vi "DataCapNew.vi"() -> ()   [LabVIEW 2022 SP3]
uses:
  b4946857-5c5e-463d-9afd-b13ad1e40e0e.vi
  37c4a671-fe09-4c27-8638-ee31c478114f.vi
  <vilib>/Analysis/baseanly.llb/Mean (DBL).vi
  <vilib>/ULx/Create Channel.llb/ULx Create Channel (AI-Voltage-Basic).vi
  <vilib>/ULx/Timing.llb/ULx Timing (Sample Clock).vi
  <vilib>/ULx/Read.llb/ULx Read (Analog 1D Wfm NChan NSamp).vi
  <vilib>/Waveform/WDTOps.llb/WDT Number of Waveform Samples DBL.vi
  <vilib>/Waveform/WDTFileIO.llb/Export Waveforms To Spreadsheet File (1D).vi
  <vilib>/Instr/_visa.llb/VISA Configure Serial Port (Instr).vi
  <vilib>/ptbypt/NI_PtbyPt.lvlib
  <vilib>/Analysis/NI_AALBase.lvlib
panel:
  out "Drag Chart":dbl(graph)
  out "Moving Average Size":dbl
  in  "sample length":i32=100
  out "Lift Chart":dbl(graph)
  out "DAQ Samples":i32
  out "DAQ Voltage Data":waveform(dbl)[](graph)
  in  "Samples":i32=-1
  in  "Sample Rate":dbl=1000.0
  in  "Manual Size":dbl
  out "Serial Samples":dbl
  in  "GoTo Angle":dbl
  out "read buffer":string
  in  "Send":bool
  in  "Period":dbl
  in  "Max Angle":dbl min=-359.9999 max=359.9999
  in  "Command":u16(ring) items=["Send Max Angle", "Send Period", "Stop Movement", "Start Movement", "Sinusoidal Motion", "Go forward", "Go backwards", "Linear Ramp", "GoTo Angle", "Set Manual Movement Size"]
  out "Angle":dbl
  in  "Port":refnum<visa-resource-name>
  out "Angle Meter":dbl(knob) scale=-100.0..100.0 scale format="%#_2f"
  out "Angle Chart":dbl(graph)
  in  "Set zero":bool
  in  "Port 2":refnum<visa-resource-name>
  out "ENC Chart 2":dbl(graph)
  out "ENC 2":dbl
  out "ENC Meter 2":dbl(knob) scale=-100.0..100.0 scale format="%#_2f"
  in  "Serial CSV Path":path
  out "Data written Serial":dbl
  out "Data written ENC":dbl
  out "Boolean 3":bool
  in  "DAQ":bool
  out "Boolean 2":bool
  in  "ENC":bool
  out "Boolean":bool
  in  "Serial":bool
  in  "STOP":bool
  # "Serial Motor Control"
  # "Serial Encoder Readout"
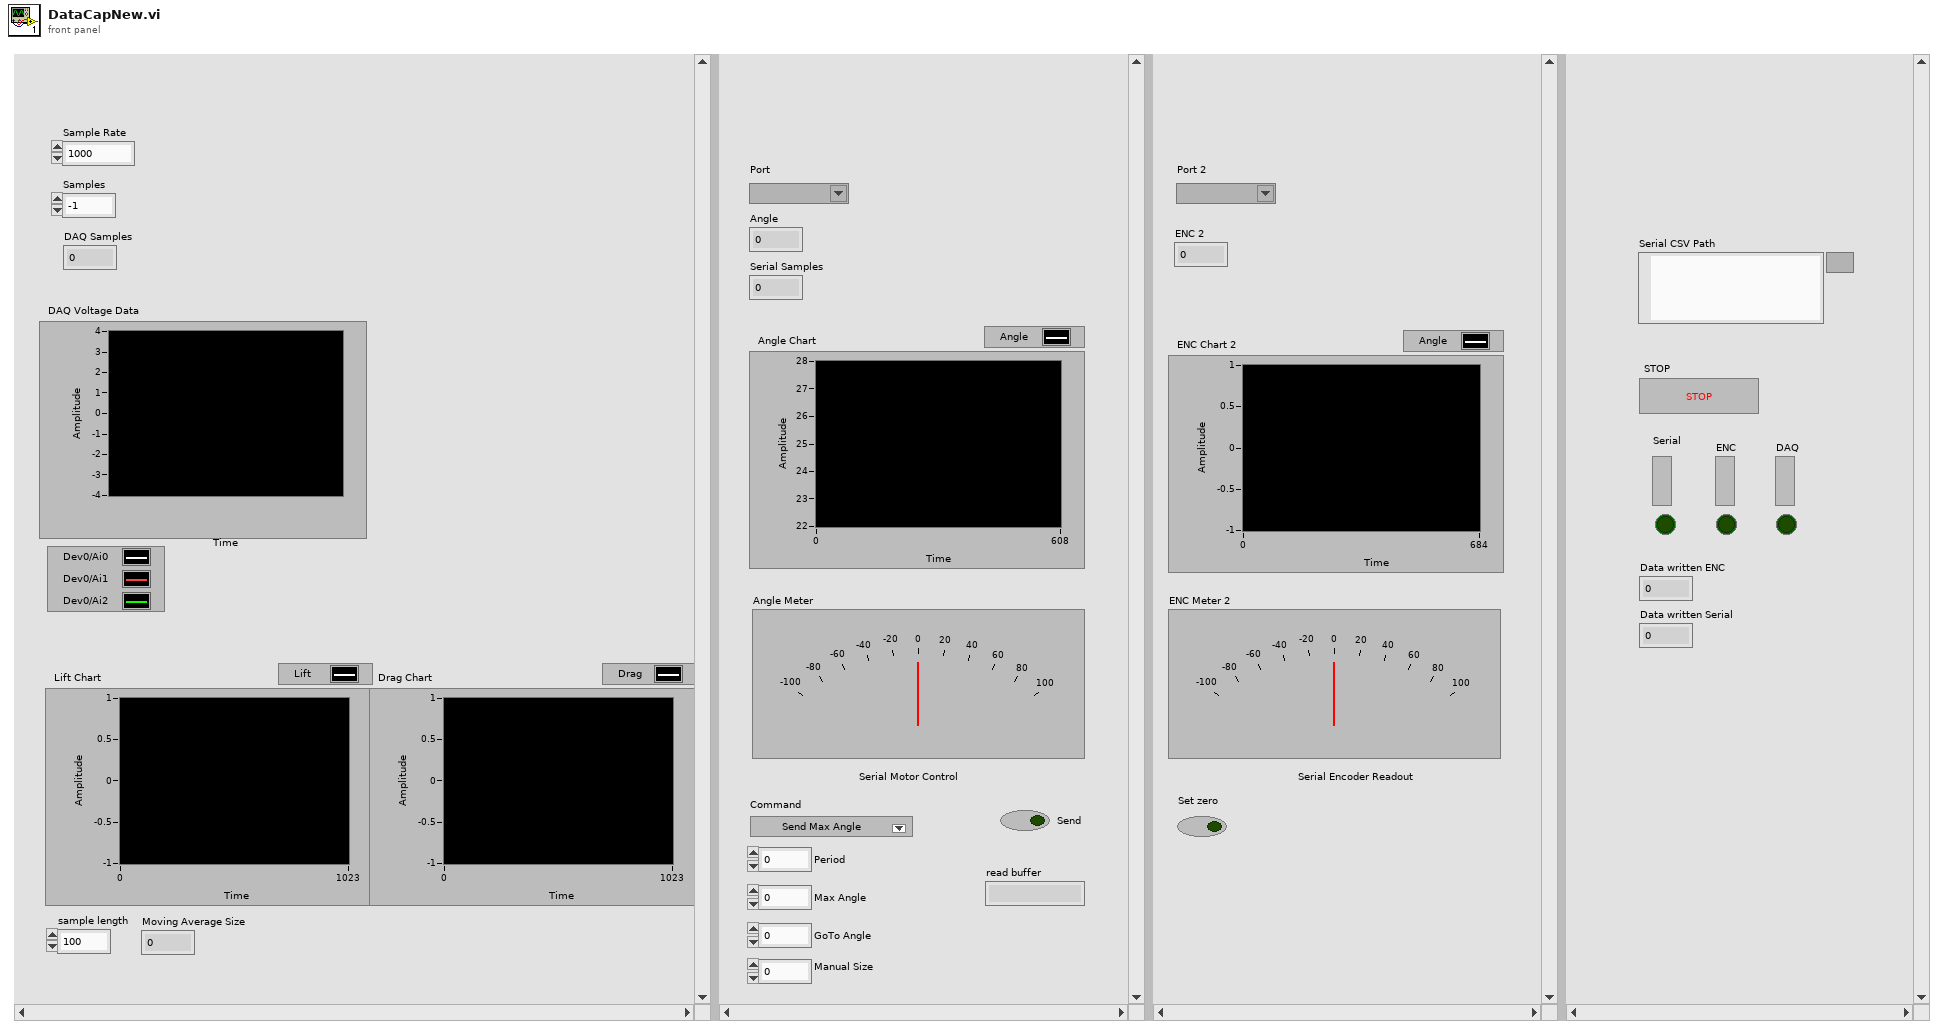
[diagram p1: front panel]
types:
  T1 = enum16{"open", "replace", "create", "open or create", "replace or create", "replace or create with confirmation"}
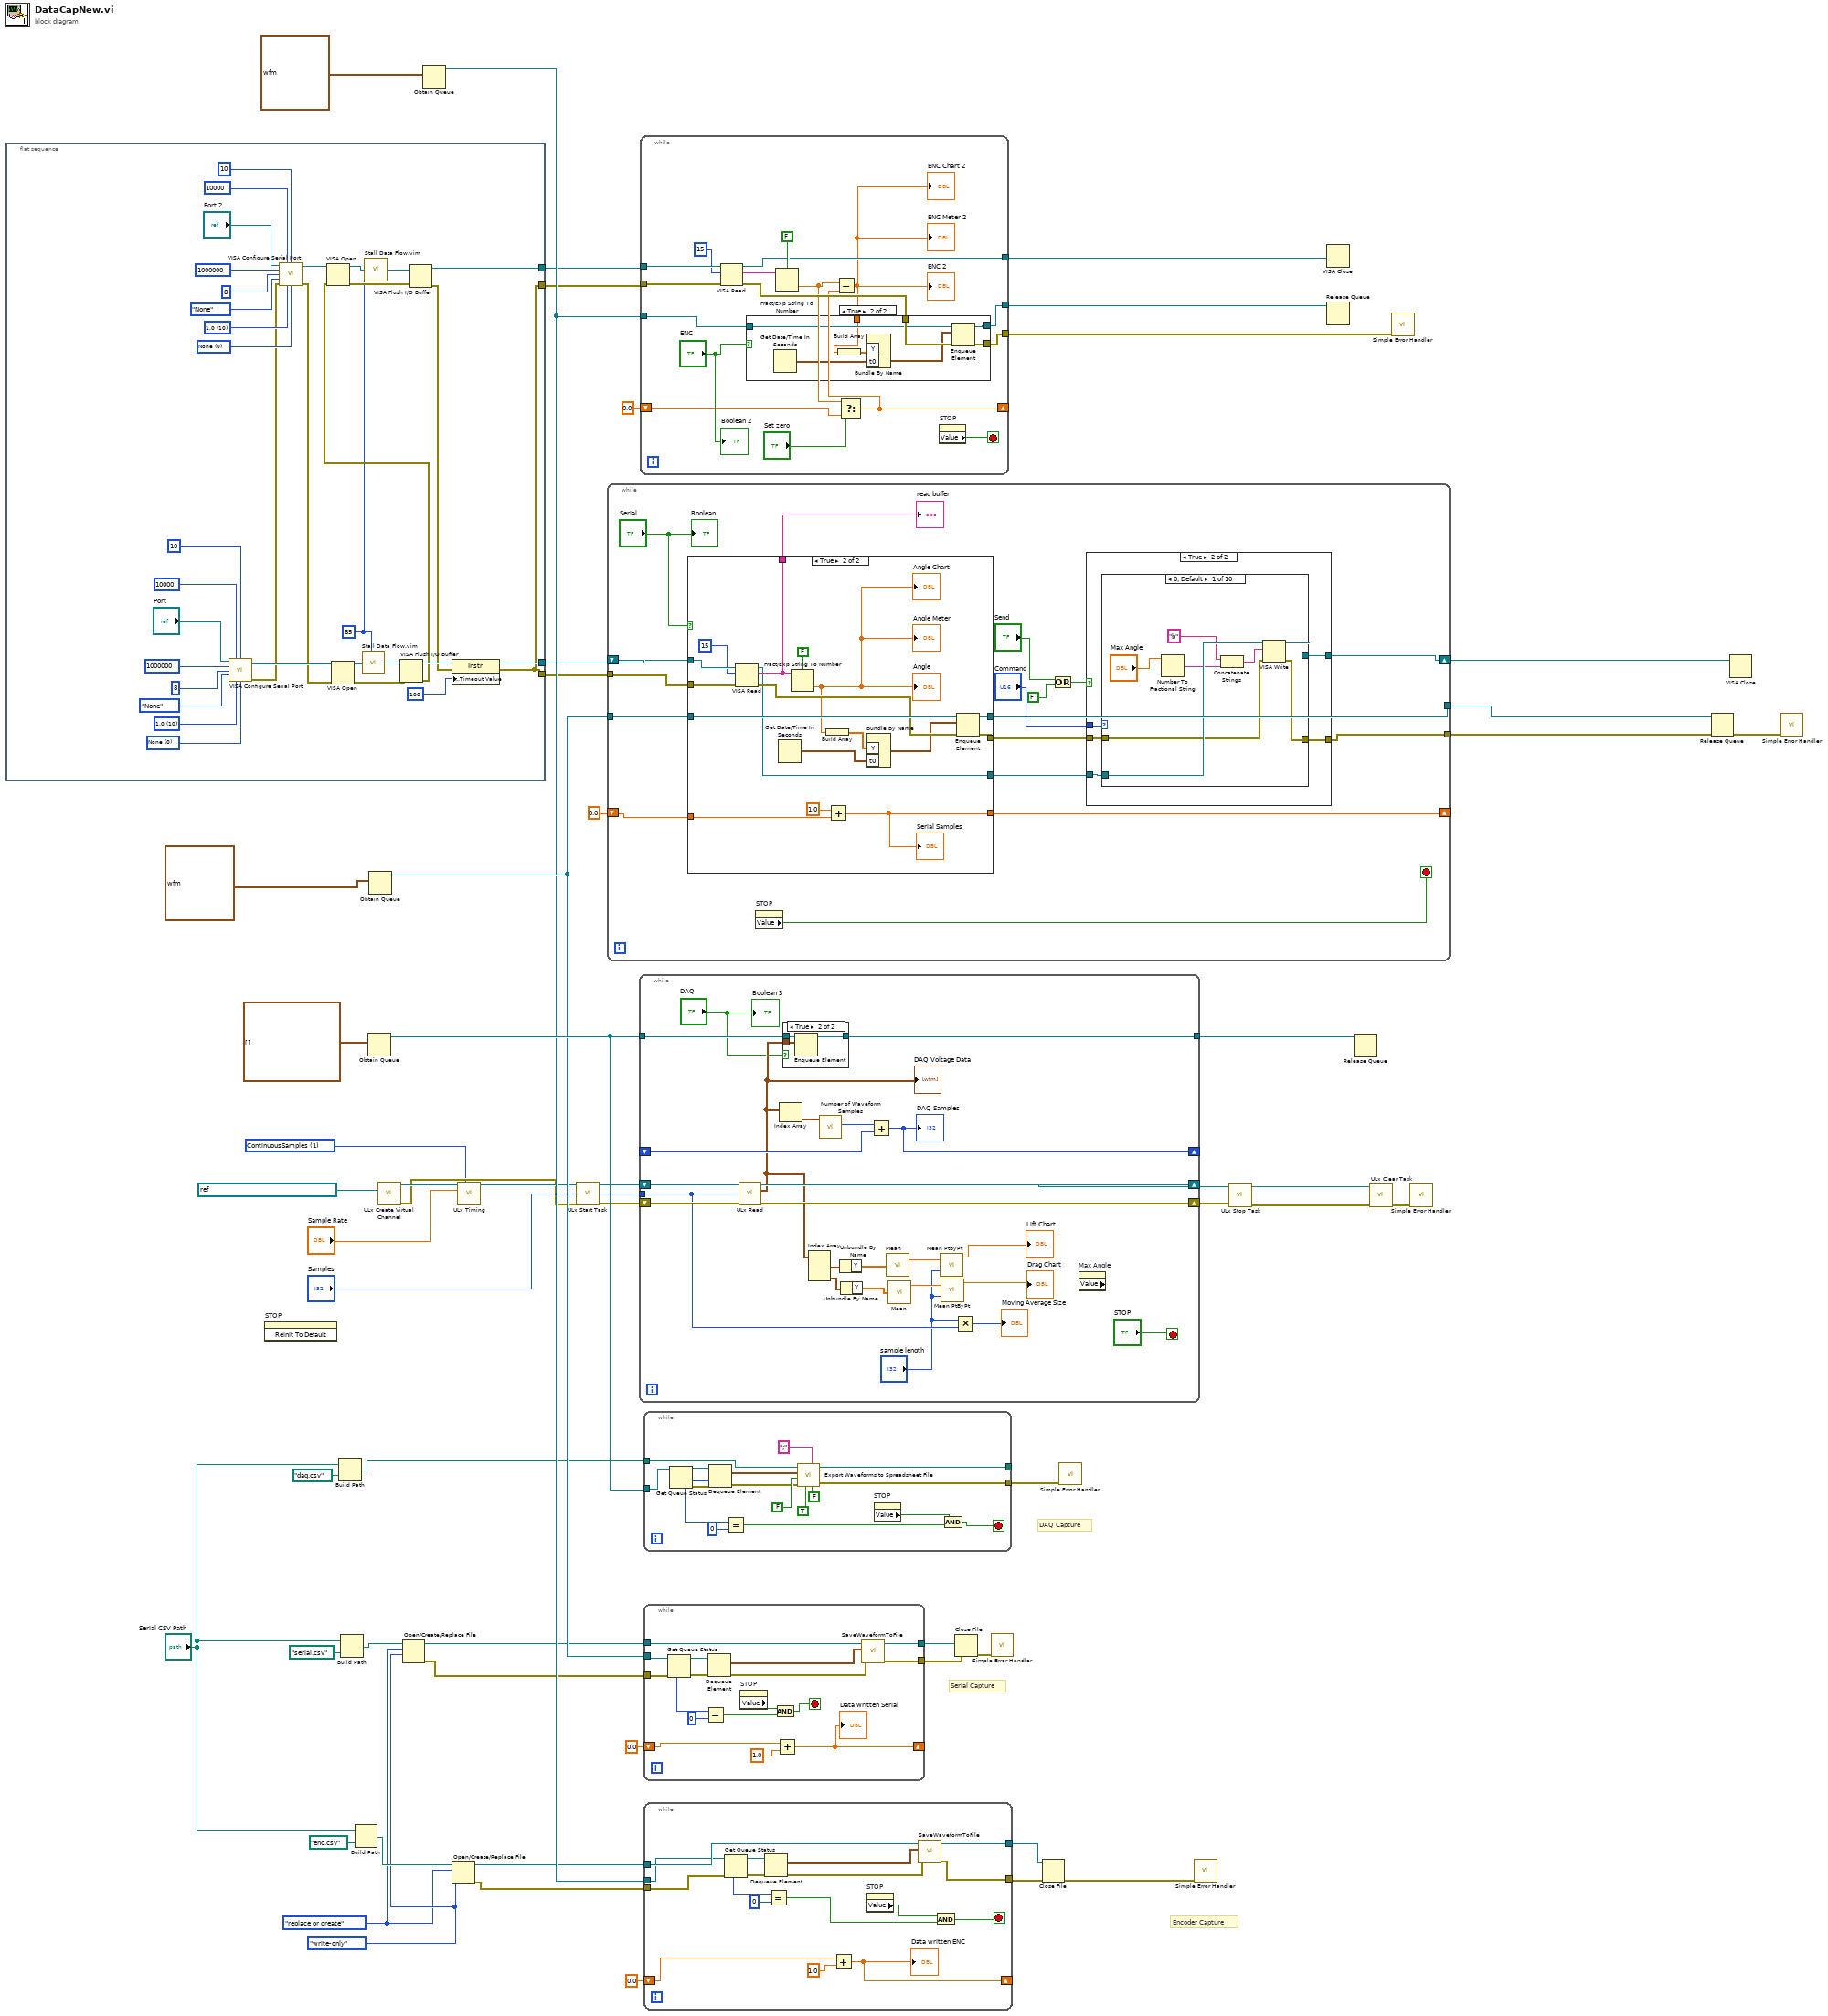
[diagram p0: block diagram]
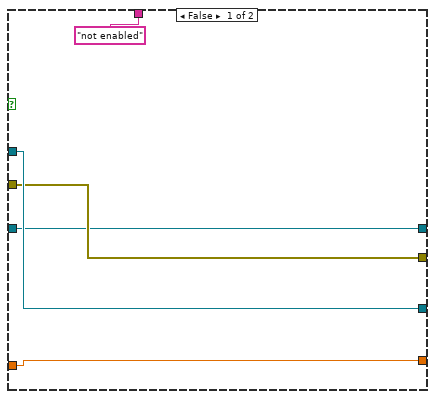
[diagram p4: hidden frame]
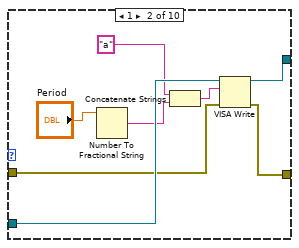
[diagram p6: hidden frame]
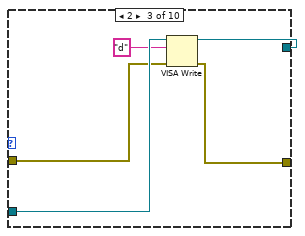
[diagram p7: hidden frame]
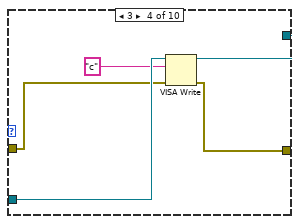
[diagram p8: hidden frame]
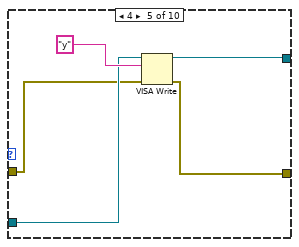
[diagram p9: hidden frame]
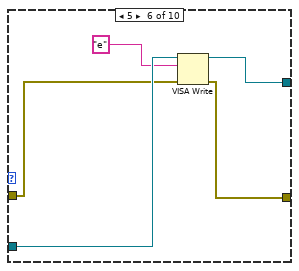
[diagram p10: hidden frame]
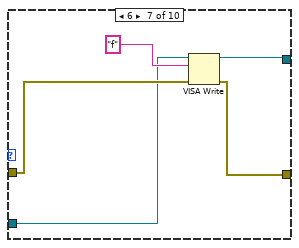
[diagram p11: hidden frame]
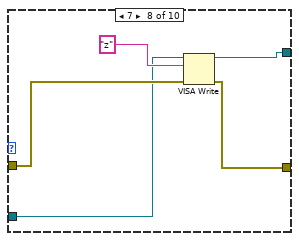
[diagram p12: hidden frame]
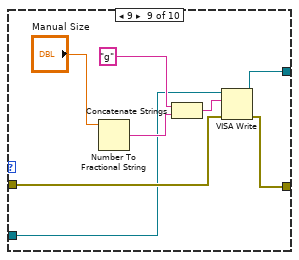
[diagram p13: hidden frame]
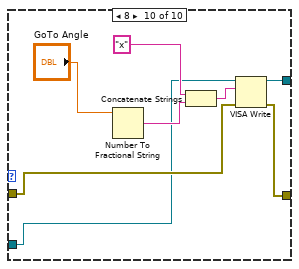
[diagram p14: hidden frame]
diagram:
  w6 = enum16{"read/write", "read-only", "write-only"}."write-only" ("access (0:read/write)")
  w5 = T1."replace or create" ("operation (0:open)")
  w33 = 1 items=["FiniteSamples", "ContinuousSamples"] ("sample mode")
  # "Encoder Capture"
  # "DAQ Capture"
  # "Serial Capture"
  n1 = flat-sequence {
    tunnel: [w72] -> w50
    tunnel: [w69] -> w49
    tunnel: [w71] -> w47
    tunnel: [w69] -> w46
    frame #0 {
      w57 = u32 85 ("milliseconds to wait")
      w76 = u16 0 items=["None", "XON/XOFF", "RTS/CTS", "XON/XOFF & RTS/CTS", "DTR/DSR", "XON/XOFF & DTR/DSR"] ("flow control (0:none)")
      w77 = u16 10 items=["1.0"=10, "1.5"=15, "2.0"=20] ("stop bits (10: 1 bit)")
      w85 = u16 0 items=["None", "XON/XOFF", "RTS/CTS", "XON/XOFF & RTS/CTS", "DTR/DSR", "XON/XOFF & DTR/DSR"] ("flow control (0:none)")
      w86 = u16 10 items=["1.0"=10, "1.5"=15, "2.0"=20] ("stop bits (10: 1 bit)")
      n2 = call-poly "VISA Configure Serial Port"("VISA resource name"="Port", "timeout (10sec)"=u32 10000, "termination char\n(0xA = '\\n' = LF)"=u8 10 ("termination char\n(0xA = '\\n' = LF)"), "baud rate (9600)"=u32 1000000, "data bits (8)"=u16 8, "parity (0:none)"=enum16{"None", "Odd", "Even", "Mark", "Space"}."None", "stop bits (10: 1 bit)"=w86, "flow control (0:none)"=w85) -> ("VISA resource name out"=w82:refnum<visa-resource-name>, "error out"=w68:errorcluster)  [unwired: 6 in]
      n3 = call-poly "VISA Configure Serial Port"("VISA resource name"="Port 2", "timeout (10sec)"=u32 10000, "termination char\n(0xA = '\\n' = LF)"=u8 10 ("termination char\n(0xA = '\\n' = LF)"), "baud rate (9600)"=u32 1000000, "data bits (8)"=u16 8, "parity (0:none)"=enum16{"None", "Odd", "Even", "Mark", "Space"}."None", "error in (no error)"=w68, "stop bits (10: 1 bit)"=w77, "flow control (0:none)"=w76) -> ("VISA resource name out"=w73:refnum<visa-resource-name>, "error out"=w67:errorcluster)  [unwired: 5 in]
      n4 = VISA Open(error in (no error)=w67, VISA resource name=w82) -> (VISA resource name=w61:refnum<visa-resource-name>, error out=w66:errorcluster)  [unwired: 3 in]
      n5 = call "Stall Data Flow.vim"("value in"=w61, "milliseconds to wait"=w57) -> ("value out"=w60:refnum<visa-resource-name>)  [unwired: 1 out]
      n6 = VISA Flush I/O Buffer(VISA resource name=w60, error in (no error)=w66) -> (VISA resource name out=w70:refnum<visa-resource-name>, error out=w65:errorcluster)  [unwired: 1 in]
      n7 = VISA Open(error in (no error)=w65, VISA resource name=w73) -> (VISA resource name=w59:refnum<visa-resource-name>, error out=w64:errorcluster)  [unwired: 3 in]
      n8 = call "Stall Data Flow.vim"("value in"=w59, "milliseconds to wait"=w57) -> ("value out"=w58:refnum<visa-resource-name>)  [unwired: 1 out]
      n9 = VISA Flush I/O Buffer(VISA resource name=w58, error in (no error)=w64) -> (VISA resource name out=w71:refnum<visa-resource-name>, error out=w62:errorcluster)  [unwired: 1 in]
      n10 = property class="Instr"(reference=w70, error in=w62, "General Settings:Timeout Value"=u32 100) -> (reference out=w72:refnum<visa-resource-name>, error out=w69:errorcluster)
    }
  }
  n11 = invoke on="STOP" class="Bool (strict)" method="Reinit To Default"() -> ()  [unwired: 3 in, 3 out]
  n12 = Build Path(base path="Serial CSV Path", name or relative path=path "daq.csv") -> (appended path=w2:path)
  n13 = Build Path(base path="Serial CSV Path", name or relative path=path "serial.csv") -> (appended path=w8:path)
  n14 = Build Path(base path="Serial CSV Path", name or relative path=path "enc.csv") -> (appended path=w10:path)
  n15 = Obtain Queue(element data type=waveform(dbl)[] []) -> (queue out=w56:refnum<queue>)  [unwired: 4 in, 2 out]
  n16 = Obtain Queue(element data type=waveform(dbl) {"t0"=timestamp(0 s since 1904-01-01), "dt"=1.0, "Y"=[]} ("Waveform")) -> (queue out=w55:refnum<queue>)  [unwired: 4 in, 2 out]
  n17 = call-poly <vilib>:"ULx Create Virtual Channel.vi"("physical channels"=refnum<k21> "Dev1/Ai0, Dev1/Ai1, Dev1/Ai2") -> ("task out"=w40:refnum<k24>, "error out"=w36:errorcluster)  [unwired: 13 in]
  n18 = Open/Create/Replace File(file path (use dialog)=w8, operation (0:open)=w5, access (0:read/write)=w6) -> (refnum out=w21:refnum<file>, error out=w20:errorcluster)  [unwired: 3 in, 1 out]
  n19 = Obtain Queue(element data type=waveform(dbl) {"t0"=timestamp(0 s since 1904-01-01), "dt"=1.0, "Y"=[]} ("Waveform")) -> (queue out=w53:refnum<queue>)  [unwired: 4 in, 2 out]
  n20 = Open/Create/Replace File(file path (use dialog)=w10, operation (0:open)=w5, access (0:read/write)=w6) -> (refnum out=w17:refnum<file>, error out=w16:errorcluster)  [unwired: 3 in, 1 out]
  n21 = call-poly <vilib>:"ULx Timing.vi"("task in"=w40, "sample mode"=w33, "rate"="Sample Rate") -> ("task out"=w38:refnum<k24>)  [unwired: 11 in, 1 out]
  n22 = call <vilib>:"ULx Start Task.vi"("task in"=w38, "error in"=w36) -> ("task out"=w37:refnum<k24>, "error out"=w35:errorcluster)  [unwired: 12 in]
  n23 = while {
    tunnel: w55 -> [w105]
    tunnel: [w97] -> w51
    tunnel: [w104] -> w52
    tunnel: w49 -> [w95]
    shift-right: [w94] -> w48
    shift-left: w50 -> [w107]
    shift-right: [w92] -> _
    shift-left: 0.0 -> [w91]
    stop <- w100 stop-if-true
    n24 = case shown="True" "Serial" {
      tunnel: w107 -> [w112 w129]
      tunnel: ["not enabled" ("read buffer") w128] -> w106
      tunnel: w105 -> [w110 w127]
      tunnel: [w110 w125] -> w104
      tunnel: [w112 w124] -> w103
      tunnel: [w111 w123] -> w98
      tunnel: w95 -> [w111 w122]
      tunnel: [w108 w117] -> w92
      tunnel: w91 -> [w108 w119]
      frame False {
      }
      frame True {
        n25 = VISA Read(VISA resource name=w129, byte count=u32 15, error in (no error)=w122) -> (VISA resource name out=w124:refnum<visa-resource-name>, read buffer=w128:string, error out=w126:errorcluster)  [unwired: 1 out]
        n26 = Get Date/Time In Seconds() -> (seconds since 1Jan1904=w115:timestamp)
        n27 = Fract/Exp String To Number(use system decimal point (T)=FALSE, string=w128) -> (number=w116:dbl)  [unwired: 2 in, 1 out]
        "Angle Chart" <- w116
        "Angle Meter" <- w116
        "Angle" <- w116
        n28 = Build Array(w116) -> (w114:dbl[])
        n29 = Add(x=1.0, y=w119) -> (x+y=w117:dbl)
        "Serial Samples" <- w117
        n30 = Bundle By Name("Y"=w114, "t0"=w115) -> (w113:waveform(dbl))  [unwired: 1 in]
        n31 = Enqueue Element(queue=w127, element=w113, error in (no error)=w126) -> (queue out=w125:refnum<queue>, error out=w123:errorcluster)  [unwired: 1 in, 1 out]
      }
    }
    "read buffer" <- w106
    n32 = property on="STOP" class="Bool (strict)"() -> ("Value"=w100:bool)  [unwired: 2 in, 2 out]
    n33 = Or(x="Send", y=FALSE) -> (x .or. y?=w101:bool)
    n34 = case shown="True" w101 {
      tunnel: "Command" -> [_ w136]
      tunnel: [w131 w135] -> w94
      tunnel: w103 -> [w131 w134]
      tunnel: w98 -> [w130 w133]
      tunnel: [w130 w132] -> w97
      frame False {
      }
      frame True {
        n35 = case shown="0, Default" w136 {
          tunnel: w134 -> [w144 w152 w157 w162 w165 w172 w173 w178 w186 w193]
          tunnel: [w143 w151 w156 w161 w166 w171 w176 w181 w185 w191] -> w135
          tunnel: w133 -> [w138 w146 w154 w159 w164 w170 w174 w179 w187 w194]
          tunnel: [w137 w145 w153 w158 w163 w169 w175 w180 w184 w192] -> w132
          frame 0, Default {
            n36 = Number To Fractional String(number="Max Angle") -> (F-format string=w140:string)  [unwired: 3 in]
            n37 = Concatenate Strings("b" ("write buffer"), w140) -> (w142:string)
            n38 = VISA Write(VISA resource name=w144, write buffer=w142, error in (no error)=w138) -> (VISA resource name out=w143:refnum<visa-resource-name>, error out=w137:errorcluster)  [unwired: 1 out]
          }
          frame 1 {
            n39 = Number To Fractional String(number="Period") -> (F-format string=w147:string)  [unwired: 3 in]
            n40 = Concatenate Strings("a" ("write buffer"), w147) -> (w150:string)
            n41 = VISA Write(VISA resource name=w152, write buffer=w150, error in (no error)=w146) -> (VISA resource name out=w151:refnum<visa-resource-name>, error out=w145:errorcluster)  [unwired: 1 out]
          }
          frame 2 {
            n42 = VISA Write(VISA resource name=w157, write buffer="d", error in (no error)=w154) -> (VISA resource name out=w156:refnum<visa-resource-name>, error out=w153:errorcluster)  [unwired: 1 out]
          }
          frame 3 {
            n43 = VISA Write(VISA resource name=w162, write buffer="c", error in (no error)=w159) -> (VISA resource name out=w161:refnum<visa-resource-name>, error out=w158:errorcluster)  [unwired: 1 out]
          }
          frame 4 {
            n44 = VISA Write(VISA resource name=w165, write buffer="y", error in (no error)=w164) -> (VISA resource name out=w166:refnum<visa-resource-name>, error out=w163:errorcluster)  [unwired: 1 out]
          }
          frame 5 {
            n45 = VISA Write(VISA resource name=w172, write buffer="e", error in (no error)=w170) -> (VISA resource name out=w171:refnum<visa-resource-name>, error out=w169:errorcluster)  [unwired: 1 out]
          }
          frame 6 {
            n46 = VISA Write(VISA resource name=w173, write buffer="f", error in (no error)=w174) -> (VISA resource name out=w176:refnum<visa-resource-name>, error out=w175:errorcluster)  [unwired: 1 out]
          }
          frame 7 {
            n47 = VISA Write(VISA resource name=w178, write buffer="z", error in (no error)=w179) -> (VISA resource name out=w181:refnum<visa-resource-name>, error out=w180:errorcluster)  [unwired: 1 out]
          }
          frame 9 {
            n48 = Number To Fractional String(number="Manual Size") -> (F-format string=w188:string)  [unwired: 3 in]
            n49 = Concatenate Strings("g" ("write buffer"), w188) -> (w190:string)
            n50 = VISA Write(VISA resource name=w186, write buffer=w190, error in (no error)=w187) -> (VISA resource name out=w185:refnum<visa-resource-name>, error out=w184:errorcluster)  [unwired: 1 out]
          }
          frame 8 {
            n51 = Number To Fractional String(number="GoTo Angle") -> (F-format string=w196:string)  [unwired: 3 in]
            n52 = Concatenate Strings("x" ("write buffer"), w196) -> (w198:string)
            n53 = VISA Write(VISA resource name=w193, write buffer=w198, error in (no error)=w194) -> (VISA resource name out=w191:refnum<visa-resource-name>, error out=w192:errorcluster)  [unwired: 1 out]
          }
        }
      }
    }
    "Boolean" <- "Serial"
  }
  n54 = while {
    tunnel: "Samples" -> [w206]
    shift-right: [w220] -> w26
    shift-left: w37 -> [w222]
    shift-right: [w219] -> w27
    shift-left: w35 -> [w221]
    shift-right: [w216] -> _
    shift-left: _ -> [w215]
    tunnel: w56 -> [w213]
    tunnel: [w212] -> w31
    stop <- "STOP" stop-if-true
    n55 = call-poly <vilib>:"ULx Read.vi"("task in"=w222, "number of samples per channel"=w206, "error in"=w221) -> ("task out"=w220:refnum<k24>, "data"=w211:waveform(dbl)[], "error out"=w219:errorcluster)  [unwired: 10 in]
    "DAQ Voltage Data" <- w211
    n56 = Index Array(array=w211) -> (element=w218:waveform(dbl))  [unwired: 1 in]
    n57 = case shown="True" "DAQ" {
      tunnel: w213 -> [w223 w226]
      tunnel: [w223 w225] -> w212
      tunnel: w211 -> [_ w224]
      frame False {
      }
      frame True {
        n58 = Enqueue Element(queue=w226, element=w224) -> (queue out=w225:refnum<queue>)  [unwired: 2 in, 2 out]
      }
    }
    n59 = Index Array(array=w211) -> (element #1=w210:waveform(dbl), element #3=w204:waveform(dbl))  [unwired: 3 in, 1 out]
    n60 = call-poly <vilib>:"Number of Waveform Samples.vi"("waveform in"=w218) -> ("number of samples"=w217:i32)  [unwired: 8 in, 2 out]
    n61 = Unbundle By Name(w210) -> ("Y"=w209:dbl[])
    n62 = Unbundle By Name(w204) -> ("Y"=w203:dbl[])
    n63 = Add(x=w217, y=w215) -> (x+y=w216:i32)
    "DAQ Samples" <- w216
    n64 = call-poly <vilib>:"Mean.vi"("X"=w209) -> ("mean"=w208:dbl)  [unwired: 1 out]
    n65 = call-poly <vilib>:"Mean.vi"("X"=w203) -> ("mean"=w202:dbl)  [unwired: 1 out]
    n66 = call <vilib>:"Mean PtByPt.vi"("x"=w208, "sample length"="sample length") -> ("mean"=→"Lift Chart":dbl)  [unwired: 2 in, 1 out]
    n67 = call <vilib>:"Mean PtByPt.vi"("x"=w202, "sample length"="sample length") -> ("mean"=→"Drag Chart":dbl)  [unwired: 2 in, 1 out]
    n68 = Multiply(x="sample length", y=w206) -> (x*y=→"Moving Average Size":i32)
    n69 = property on="Max Angle" class="DigNum (strict)" props=["Value"]() -> ()  [unwired: 2 in, 3 out]
    "Boolean 3" <- "DAQ"
  }
  n70 = while {
    tunnel: w47 -> [w243]
    tunnel: w46 -> [w242]
    tunnel: [w237] -> w45
    tunnel: [w236] -> w44
    tunnel: w53 -> [w234]
    tunnel: [w233] -> w43
    shift-right: [w231] -> _
    shift-left: 0.0 -> [w228]
    stop <- w235 stop-if-true
    n71 = VISA Read(VISA resource name=w243, byte count=u32 15, error in (no error)=w242) -> (VISA resource name out=w233:refnum<visa-resource-name>, read buffer=w240:string, error out=w238:errorcluster)  [unwired: 1 out]
    n72 = Fract/Exp String To Number(use system decimal point (T)=FALSE, string=w240) -> (number=w229:dbl)  [unwired: 2 in, 1 out]
    n73 = Select(t=w229, s="Set zero", f=w228) -> (s? t:f=w231:dbl)
    n74 = Subtract(x=w229, y=w231) -> (x-y=w230:dbl)
    "ENC Chart 2" <- w230
    "ENC Meter 2" <- w230
    "ENC 2" <- w230
    n75 = case shown="True" "ENC" {
      tunnel: w238 -> [w244 w251]
      tunnel: [w244 w250] -> w237
      tunnel: [w245 w249] -> w236
      tunnel: w234 -> [w245 w248]
      tunnel: w230 -> [_ w247]
      frame False {
      }
      frame True {
        n76 = Get Date/Time In Seconds() -> (seconds since 1Jan1904=w252:timestamp)
        n77 = Build Array(w247) -> (w253:dbl[])
        n78 = Bundle By Name("Y"=w253, "t0"=w252) -> (w246:waveform(dbl))  [unwired: 1 in]
        n79 = Enqueue Element(queue=w248, element=w246, error in (no error)=w251) -> (queue out=w249:refnum<queue>, error out=w250:errorcluster)  [unwired: 1 in, 1 out]
      }
    }
    n80 = property on="STOP" class="Bool (strict)"() -> ("Value"=w235:bool)  [unwired: 2 in, 2 out]
    "Boolean 2" <- "ENC"
  }
  n81 = while {
    tunnel: w56 -> [w269]
    tunnel: [w258] -> w1
    tunnel: [w257] -> _
    tunnel: w2 -> [w255]
    stop <- w265 stop-if-true
    n82 = Get Queue Status(queue=w269) -> (queue out=w263:refnum<queue>, # pending insert=w271:i32, error out=w270:errorcluster, # elements in queue=w267:i32)  [unwired: 2 in, 4 out]
    n83 = Dequeue Element(queue=w263, timeout in ms (-1)=w271, error in (no error)=w270) -> (element=w261:waveform(dbl)[], error out=w259:errorcluster)  [unwired: 2 out]
    n84 = Equal?(x=w267, y=0) -> (x = y?=w264:bool)
    n85 = call-poly <vilib>:"Export Waveforms to Spreadsheet File.vi"("header? (write header:T)"=FALSE, "delimiter (Tab)"=";", "append to file? (new file:F)"=TRUE, "error in (no error)"=w259, "multiple time columns? (single:F)"=FALSE ("header? (write header:T)"), "waveforms"=w261, "file path (dialog if empty)"=w255) -> ("error out"=w258:errorcluster, "new file path (Not A Path if cancelled)"=w257:path)  [unwired: 3 in]
    n86 = property on="STOP" class="Bool (strict)"() -> ("Value"=w266:bool)  [unwired: 2 in, 2 out]
    n87 = And(x=w266, y=w264) -> (x .and. y?=w265:bool)
  }
  n88 = while {
    tunnel: w55 -> [w286]
    tunnel: [w283] -> w19
    tunnel: w20 -> [w280]
    tunnel: w21 -> [w281]
    tunnel: [w282] -> w22
    shift-right: [w274] -> _
    shift-left: 0.0 -> [w273]
    stop <- w277 stop-if-true
    n89 = Get Queue Status(queue=w286, error in (no error)=w280) -> (queue out=w288:refnum<queue>, error out=w287:errorcluster, # elements in queue=w279:i32)  [unwired: 1 in, 5 out]
    n90 = Equal?(x=w279, y=0) -> (x = y?=w275:bool)
    n91 = Dequeue Element(queue=w288, error in (no error)=w287) -> (element=w285:waveform(dbl), error out=w284:errorcluster)  [unwired: 1 in, 2 out]
    n92 = property on="STOP" class="Bool (strict)"() -> ("Value"=w276:bool)  [unwired: 2 in, 2 out]
    n93 = And(x=w276, y=w275) -> (x .and. y?=w277:bool)
    n94 = Add(x=w273, y=1.0) -> (x+y=w274:dbl)
    "Data written Serial" <- w274
    n95 = call "SaveWaveformToFile.vi"("error in (no error)"=w284, "Waveform"=w285, "Byte Stream File in"=w281) -> ("error out"=w283:errorcluster, "Byte Stream File out"=w282:refnum<file>)  [unwired: 7 in]
  }
  n96 = while {
    tunnel: w53 -> [w292]
    tunnel: [w297] -> w14
    tunnel: w17 -> [w296]
    tunnel: w16 -> [w295]
    tunnel: [w294] -> w13
    shift-right: [w290] -> _
    shift-left: 0.0 -> [w289]
    stop <- w298 stop-if-true
    n97 = Get Queue Status(queue=w292, error in (no error)=w295) -> (queue out=w305:refnum<queue>, error out=w304:errorcluster, # elements in queue=w301:i32)  [unwired: 1 in, 5 out]
    n98 = Dequeue Element(queue=w305, error in (no error)=w304) -> (element=w303:waveform(dbl), error out=w302:errorcluster)  [unwired: 1 in, 2 out]
    n99 = Equal?(x=w301, y=0) -> (x = y?=w299:bool)
    n100 = Add(x=w289, y=1.0) -> (x+y=w290:dbl)
    "Data written ENC" <- w290
    n101 = property on="STOP" class="Bool (strict)"() -> ("Value"=w293:bool)  [unwired: 2 in, 2 out]
    n102 = call "SaveWaveformToFile.vi"("error in (no error)"=w302, "Waveform"=w303, "Byte Stream File in"=w296) -> ("error out"=w297:errorcluster, "Byte Stream File out"=w294:refnum<file>)  [unwired: 7 in]
    n103 = And(x=w293, y=w299) -> (x .and. y?=w298:bool)
  }
  n104 = Close File(refnum=w22, error in=w19) -> (error out=w18:errorcluster)  [unwired: 1 out]
  n105 = call <vilib>:"Simple Error Handler.vi"("error in (no error)"=w18) -> ()  [unwired: 4 in, 5 out]
  n106 = Close File(refnum=w13, error in=w14) -> (error out=w15:errorcluster)  [unwired: 1 out]
  n107 = call <vilib>:"Simple Error Handler.vi"("error in (no error)"=w1) -> ()  [unwired: 4 in, 5 out]
  n108 = call <vilib>:"Simple Error Handler.vi"("error in (no error)"=w15) -> ()  [unwired: 4 in, 5 out]
  n109 = call <vilib>:"ULx Stop Task.vi"("error in"=w27, "task in"=w26) -> ("error out"=w29:errorcluster, "task out"=w30:refnum<k24>)  [unwired: 8 in]
  n110 = VISA Close(VISA resource name=w43) -> ()  [unwired: 1 in, 1 out]
  n111 = Release Queue(queue=w44) -> ()  [unwired: 2 in, 3 out]
  n112 = Release Queue(queue=w31) -> ()  [unwired: 2 in, 3 out]
  n113 = call <vilib>:"ULx Clear Task.vi"("task in"=w30, "error in"=w29) -> ("error out"=w28:errorcluster)  [unwired: 13 in]
  n114 = call <vilib>:"Simple Error Handler.vi"("error in (no error)"=w45) -> ()  [unwired: 4 in, 5 out]
  n115 = call <vilib>:"Simple Error Handler.vi"("error in (no error)"=w28) -> ()  [unwired: 4 in, 5 out]
  n116 = Release Queue(queue=w52, error in (no error)=w51) -> (error out=w54:errorcluster)  [unwired: 1 in, 2 out]
  n117 = VISA Close(VISA resource name=w48) -> ()  [unwired: 1 in, 1 out]
  n118 = call <vilib>:"Simple Error Handler.vi"("error in (no error)"=w54) -> ()  [unwired: 4 in, 5 out]
